vi "ExecuteOffensivePlay_v2.vi"(0 "object in":refnum<class "Game.lvclass">, 5 "error in (no error)":errorcluster) -> (14 "object out":refnum<class "Game.lvclass">, 19 "error out":errorcluster)   [LabVIEW 2023, in "Game.lvclass"]
uses:
  Game.lvclass
  Game.lvclass/Game.ctl
  Team_class/Team.lvclass/Team.ctl
  Team_class/Read RobotRef.vi
  Team_class/Write RobotRef.vi
  Ally_class/Ally.lvclass
  C:/Users/ebert/Documents/codes/SSL/repo/SSL_AI/Team_class/Team.lvclass
  Robot_class/Robot.lvclass
  NewSTP/NewPlays/Play_v2_class/Play_v2.lvclass
  NewSTP/Playbook_v2_class/Playbook_v2.lvclass
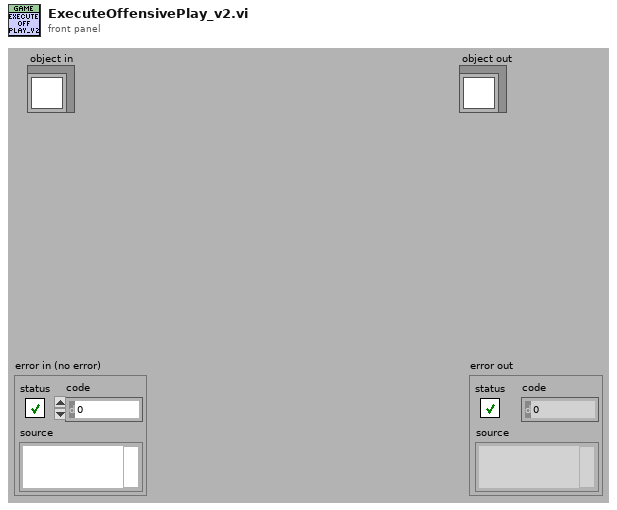
[diagram p1: front panel]
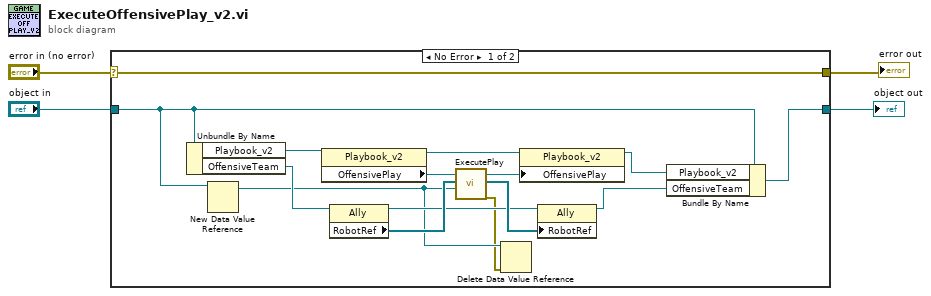
[diagram p0: block diagram]
diagram:
  n1 = case shown="No Error" "error in (no error)" {
    selector: "error in (no error)" -> [w19 w21]
    tunnel: [w19 w21] -> w3
    tunnel: [w8 w20] -> w1
    tunnel: "object in" -> [w7 w20]
    frame No Error {
      n2 = Unbundle By Name(w7) -> ("Playbook_v2"=w18:refnum<class "Playbook_v2.lvclass">, "OffensiveTeam"=w16:refnum<class "Ally.lvclass">)
      n3 = New Data Value Reference(data value=w7) -> (data value reference=w6:refnum<data-value>)  [unwired: 1 in, 1 out]
      n4 = property class="Playbook_v2"(reference=w18) -> (reference out=w12:refnum<class "Playbook_v2.lvclass">, "OffensivePlay"=w17:refnum<class "Play_v2.lvclass">)  [unwired: 1 in, 1 out]
      n5 = property class="Ally"(reference=w16) -> (reference out=w13:refnum<class "Ally.lvclass">, "RobotRef"=w15:refnum<class "Robot.lvclass">[])  [unwired: 1 in, 1 out]
      n6 = call-dynamic "ExecutePlay.vi"("object in"=w17, "Robots in"=w15, "GameRef"=w6) -> ("object out"=w11:refnum<class "Play_v2.lvclass">, "Robots out"=w14:refnum<class "Robot.lvclass">[], "error out"=w5:errorcluster)  [unwired: 14 in]
      n7 = Delete Data Value Reference(data value reference=w6, error in=w5) -> ()  [unwired: 2 out]
      n8 = property class="Playbook_v2"(reference=w12, "OffensivePlay"=w11) -> (reference out=w10:refnum<class "Playbook_v2.lvclass">)  [unwired: 1 in, 1 out]
      n9 = property class="Ally"(reference=w13, "RobotRef"=w14) -> (reference out=w9:refnum<class "Ally.lvclass">)  [unwired: 1 in, 1 out]
      n10 = Bundle By Name(cluster=w7, "Playbook_v2"=w10, "OffensiveTeam"=w9) -> (w8:refnum<class "Game.lvclass">)
    }
    frame Error {
    }
  }
  "error out" <- w3
  "object out" <- w1
